vi "Blob ReadData_SGL.vi"(8 "error in (no error)":errorcluster, 11 "Blob in":refnum<class "Blob.lvclass">) -> (0 "error out":errorcluster, 2 "NCHW Blob":sgl[][][][](array[numeric]), 3 "Blob out":refnum<class "Blob.lvclass">)   [LabVIEW 2020, in "OpenLvVision_OpenCv.lvlib" / "Blob.lvclass"]
doc: "Retruns the data that is stored as nchw array inside the blob."
uses:
  Blob.lvclass
  C:/Users/lukas/Downloads/OpenLvVision_OpenCv/SourceCode/LabView/OpenLvVision_OpenCv/_LvHelpers/EdvrObject/EdvrObject.lvclass
  _LvHelpers/EdvrObject/EdvrObject.lvclass/EdvrObject.ctl
  _LvHelpers/EdvrObject/EdvrObject.lvclass
  Dlls/OlvOpenCvWrapper.dll
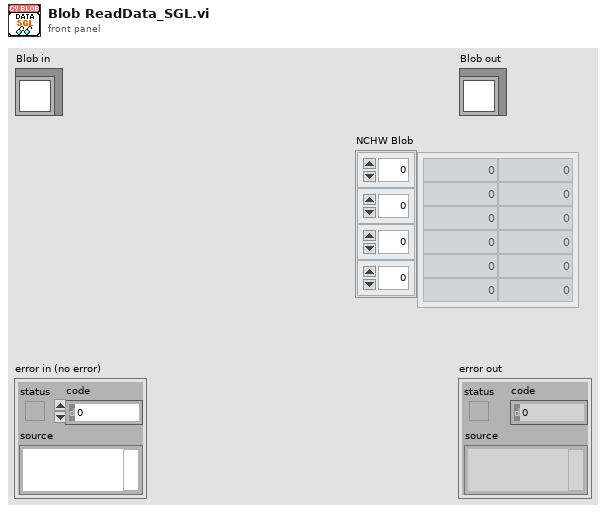
[diagram p1: front panel]
types:
  T1 = typedef "OpenLvVision_OpenCv.lvlib/EdvrObject.lvclass/Edvr.ctl" = refnum<data-value>
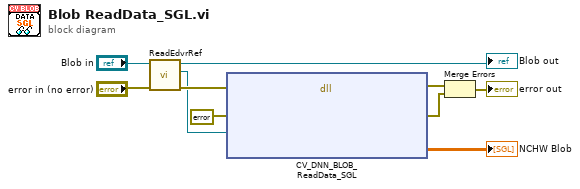
[diagram p0: block diagram]
diagram:
  n1 = call "ReadEdvrRef.vi"("error in (no error)"="error in (no error)", "EdvrObject in"="Blob in") -> ("error out"=w10:errorcluster, "Edvr"=w4:T1, "EdvrObject out"=→"Blob out":refnum<class "Blob.lvclass">)  [unwired: 7 in]
  n2 = dll-call lib="C:/Users/lukas/Downloads/OpenLvVision_OpenCv/SourceCode/LabView/OpenLvVision_OpenCv/Dlls/OlvOpenCvWrapper.dll" fn="CV_DNN_BLOB_ReadData_SGL"(error in=w10, "Error"=errorcluster {"status"=FALSE, "code"=0, "source"=""} ("error out"), "edvrRef"=w4) -> (error out=w8:errorcluster, "Error"=w7:errorcluster, "nchwArrayHandle"=→"NCHW Blob":sgl[][][][])  [unwired: 5 in, 1 out]
  n3 = Merge Errors(w8, w7) -> (→"error out":errorcluster)
